vi "Append Dictionary Element.vi"(8 "error in (no error)":errorcluster, 9 "value":variant, 10 "key":string, 11 "Control Experiment in":refnum<class "Control Experiment SM.lvclass">) -> (0 "error out":errorcluster, 3 "Control Experiment out":refnum<class "Control Experiment SM.lvclass">)   [LabVIEW 2016, in "Control Experiment SM.lvclass"]
uses:
  Control Experiment SM.lvclass
  Control Experiment SM.lvclass/Control Experiment SM.ctl
  <userlib>/_OpenG.lib/dictionary/dictionary.llb/Dictionary Update (by scalar value)__ogtk.vi
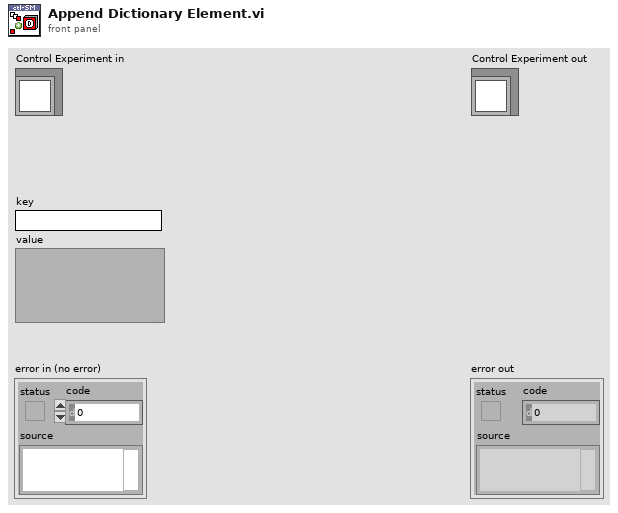
[diagram p1: front panel]
types:
  T1 = typedef "Dictionary Object RefNum__ogtk.ctl" = refnum<k1>
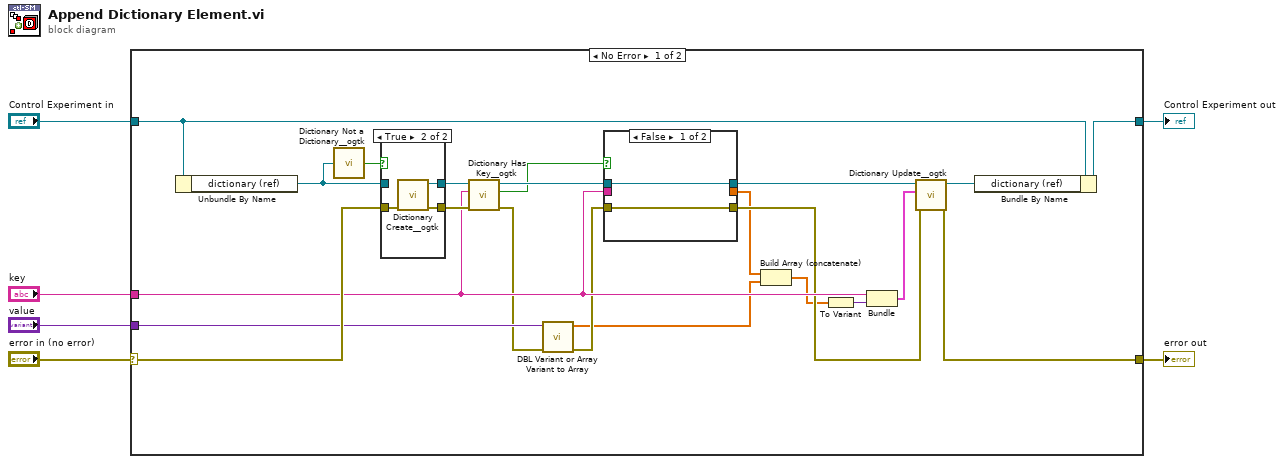
[diagram p0: block diagram]
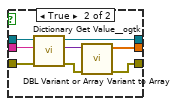
[diagram p3: hidden frame]
diagram:
  n1 = case shown="No Error" "error in (no error)" {
    selector: "error in (no error)" -> [w23 w44]
    tunnel: [w25 w44] -> w5
    tunnel: [w28 w45] -> w3
    tunnel: "Control Experiment in" -> [w27 w45]
    tunnel: "key" -> [w16 _]
    tunnel: "value" -> [w12 _]
    frame No Error {
      n2 = Unbundle By Name(w27) -> ("dictionary (ref)"=w22:T1)
      n3 = call <userlib>:"Dictionary Not a Dictionary__ogtk.vi"("dictionary"=w22) -> ("not a dictionary?"=w24:bool)
      n4 = case shown="True" w24 {
        tunnel: [w30 w33] -> w21
        tunnel: w22 -> [w30 _]
        tunnel: [w29 w32] -> w20
        tunnel: w23 -> [w29 w31]
        frame False {
        }
        frame True {
          n5 = call <userlib>:"Dictionary Create__ogtk.vi"("error in (no error)"=w31) -> ("error out"=w32:errorcluster, "dictionary out"=w33:T1)  [unwired: 9 in]
        }
      }
      n6 = call <userlib>:"Dictionary Has Key__ogtk.vi"("error in (no error)"=w20, "key"=w16, "dictionary"=w21) -> ("error out"=w11:errorcluster, "Has Key?"=w15:bool, "dictionary out"=w19:T1)  [unwired: 6 in]
      n7 = call "DBL Variant or Array Variant to Array.vi"("error in (no error)"=w11, "value"=w12) -> ("error out"=w10:errorcluster, "Array"=w9:dbl[])  [unwired: 8 in]
      n8 = case shown="False" w15 {
        tunnel: w19 -> [w34 w43]
        tunnel: w10 -> [w35 w42]
        tunnel: w16 -> [_ w41]
        tunnel: [w35 w37] -> w14
        tunnel: [w34 w40] -> w13
        tunnel: [_ w36] -> w8
        frame False {
        }
        frame True {
          n9 = call <userlib>:"Dictionary Get Value__ogtk.vi"("error in"=w42, "key"=w41, "dictionary"=w43) -> ("error out"=w38:errorcluster, "value"=w39:variant, "dictionary out"=w40:T1)  [unwired: 5 in, 1 out]
          n10 = call "DBL Variant or Array Variant to Array.vi"("error in (no error)"=w38, "value"=w39) -> ("error out"=w37:errorcluster, "Array"=w36:dbl[])  [unwired: 8 in]
        }
      }
      n11 = Build Array (concatenate)(w8, w9) -> (w7:dbl[])
      n12 = To Variant(anything=w7) -> (Variant=w17:variant)
      n13 = Bundle("key"=w16, "Variant"=w17) -> (w18:cluster{"key":string, "Variant":variant})  [unwired: 1 in]
      n14 = call-poly <userlib>:"Dictionary Update__ogtk.vi"("error in (no error)"=w14, "key-value"=w18, "dictionary"=w13) -> ("error out"=w25:errorcluster, "dictionary out"=w26:T1)  [unwired: 6 in, 1 out]
      n15 = Bundle By Name(cluster=w27, "dictionary (ref)"=w26) -> (w28:refnum<class "Control Experiment SM.lvclass">)
    }
    frame Error {
    }
  }
  "error out" <- w5
  "Control Experiment out" <- w3
